vi "Clock.vi"(11 "Slices":u32) -> (3 "Clk":bool)   [LabVIEW 2012]
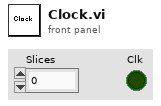
[diagram p1: front panel]
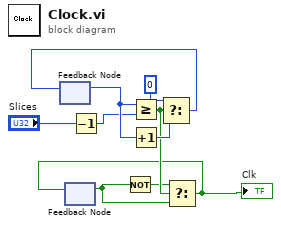
[diagram p0: block diagram]
diagram:
  n1 = feedback #1() -> (w9:i32)  [unwired: 1 in]
  n2 = feedback #2() -> (w3:bool)  [unwired: 1 in]
  n3 = Decrement(x="Slices") -> (x-1=w1:u32)
  n4 = Not(x=w3) -> (.not. x?=w4:bool)
  n5 = Greater Or Equal?(x=w9, y=w1) -> (x >= y?=w6:bool)
  n6 = Increment(x=w9) -> (x+1=w8:i32)
  n7 = Select(t=0, s=w6, f=w8) -> (s? t:f=w7:i32)
  n8 = feedback-in #1(w7) -> ()
  n9 = Select(t=w4, s=w6, f=w3) -> (s? t:f=w5:bool)
  "Clk" <- w5
  n10 = feedback-in #2(w5) -> ()
